vi "Window call-Live Imaging.vi"(8 "error in (no error)":errorcluster, 11 "UI ctrl refs":T1) -> (0 "error out":errorcluster)   [LabVIEW 2013]
uses:
  Typedefs/UI ctrl refs cluster.ctl
  Typedefs/Laser control knob.ctl
  Typedefs/Frame Size.ctl
  Typedefs/Plane Mode.ctl
  Typedefs/PMT control knob.ctl
  Global Variables/General Globals.vi
panel:
  in  "Live imaging window name":string="Live Imaging Window.vi"
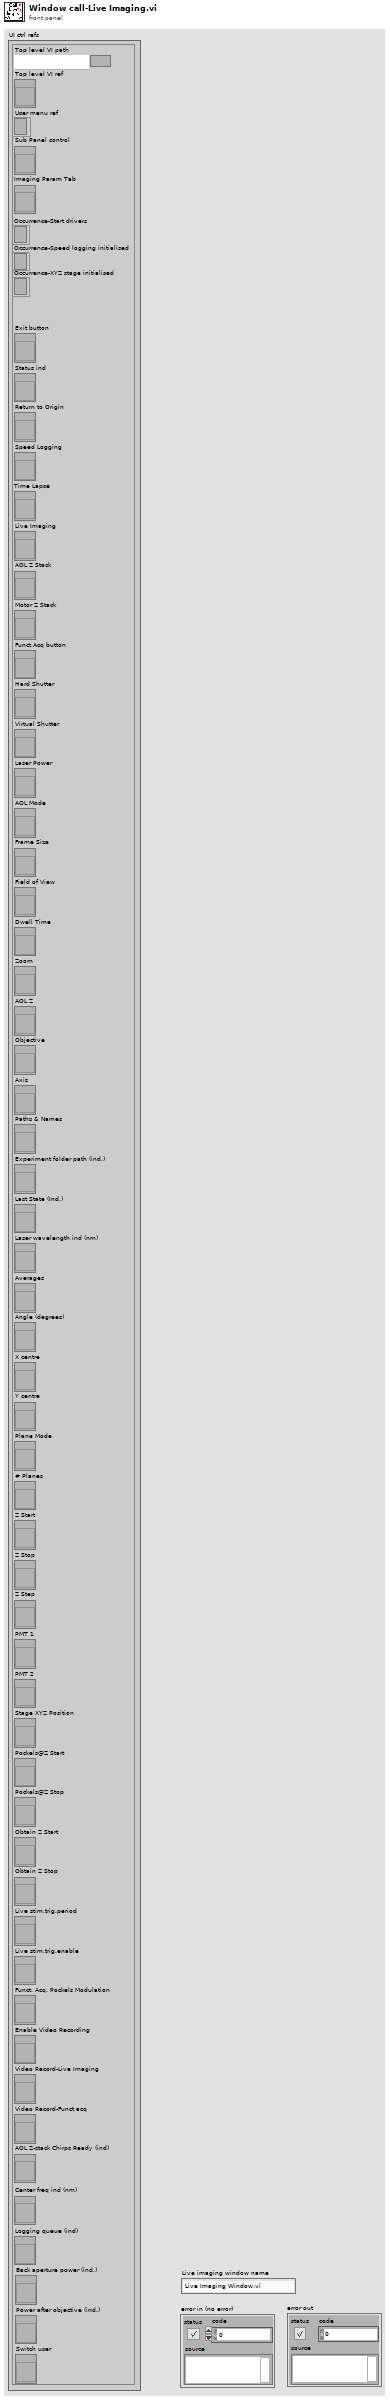
[diagram p1: front panel]
types:
  T1 = typedef "UI ctrl refs cluster.ctl" = cluster{"Top level VI path":path, "Top level VI ref":refnum<vi>, "User menu ref":refnum<k9>, "Sub Panel control":refnum<vi>, "Imaging Param Tab":refnum<vi>, "Occurrence-Start drivers":refnum<k4>, "Occurrence-Speed logging initialised":refnum<k4>, "Occurrence-XYZ stage initialised":refnum<k4>, "Exit button":refnum<vi>, "Status ind":refnum<vi>, "Return to Origin":refnum<vi>, "Speed Logging":refnum<vi>, "Time Lapse":refnum<vi>, "Live Imaging":refnum<vi>, "AOL Z Stack":refnum<vi>, "Motor Z Stack":refnum<vi>, "Funct Acq button":refnum<vi>, "Hard Shutter":refnum<vi>, "Virtual Shutter":refnum<vi>, "Laser Power":refnum<vi>, "AOL Mode":refnum<vi>, "Frame Size":refnum<vi>, "Field of View":refnum<vi>, "Dwell Time":refnum<vi>, "Zoom":refnum<vi>, "AOL Z":refnum<vi>, "Objective":refnum<vi>, "Axis":refnum<vi>, "Paths & Names":refnum<vi>, "Experiment folder path (ind.)":refnum<vi>, "Last State (Ind.)":refnum<vi>, "Laser wavelength ind (nm)":refnum<vi>, "Averages":refnum<vi>, "Angle (degrees)":refnum<vi>, "X centre":refnum<vi>, "Y centre":refnum<vi>, "Plane Mode":refnum<vi>, "# Planes":refnum<vi>, "Z Start":refnum<vi>, "Z Stop":refnum<vi>, "Z Step":refnum<vi>, "PMT 1":refnum<vi>, "PMT 2":refnum<vi>, "Stage XYZ Position":refnum<vi>, "Pockels@Z Start":refnum<vi>, "Pockels@Z Stop":refnum<vi>, "Obtain Z Start":refnum<vi>, "Obtain Z Stop":refnum<vi>, "Live stim.trig.period":refnum<vi>, "Live stim.trig.enable":refnum<vi>, "Funct. Acq. Pockels Modulation":refnum<vi>, "Enable Video Recording":refnum<vi>, "Video Record-Live Imaging":refnum<vi>, "Video Record-Funct acq":refnum<vi>, "AOL Z-stack Chirps Ready (ind)":refnum<vi>, "Center freq ind (nm)":refnum<vi>, "Logging queue (ind)":refnum<vi>, "Back aperture power (ind.)":refnum<vi>, "Power after objective (ind.)":refnum<vi>, "Switch user":refnum<vi>}
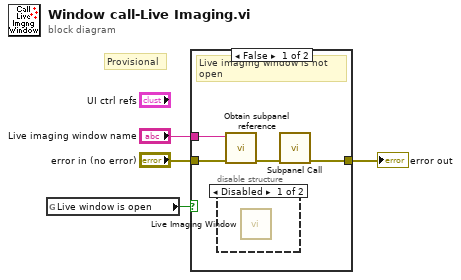
[diagram p0: block diagram]
diagram:
  # "Provisional"
  n1 = global read "General Globals.vi" "Live window is open"() -> (w3:bool)
  n2 = case shown="False" w3 {
    tunnel: "error in (no error)" -> [w7 w9]
    tunnel: [w8 w9] -> w2
    tunnel: "Live imaging window name" -> [w5 _]
    frame False {
      # "Live imaging window is not open"
      n3 = disable-structure shown="Disabled" {
        frame Disabled {
          n4 = call "Live Imaging Window.vi"() -> ()  [unwired: 12 in]
        }
        frame Enabled {
        }
      }
      n5 = call "Obtain subpanel reference.vi"("error in (no error)"=w7, "Subpanel VI name (plus \".vi\" file extension)"=w5) -> ("error out"=w6:errorcluster)  [unwired: 8 in, 1 out]
      n6 = call "Subpanel Call.vi"("error in (no error)"=w6) -> ("error out"=w8:errorcluster)  [unwired: 10 in]
    }
    frame True {
      # "Live imaging window is already open"
    }
  }
  "error out" <- w2
